vi "tiffU16to2xU8.vi"(10 "U16":u16[][](array[numeric])) -> (2 "Bytes":u8[](array[numeric]))   [LabVIEW 2017, in "LVTiffWriter.lvlib"]
uses:
  LVTiffWriter.lvlib
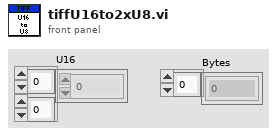
[diagram p1: front panel]
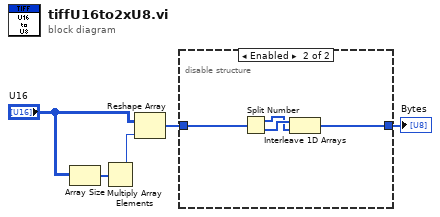
[diagram p0: block diagram]
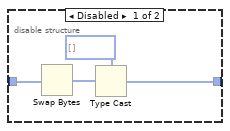
[diagram p2: hidden frame]
diagram:
  n1 = Array Size(array="U16") -> (size(s)=w2:i32[])
  n2 = Multiply Array Elements(1:w2) -> (0:w3:i32)
  n3 = Reshape Array("U16", w3) -> (w1:u16[])
  n4 = disable-structure shown="Enabled" {
    disable-tunnel: [w8 w10] -> w4
    disable-tunnel: w1 -> [w7 w11]
    frame Disabled {
      n5 = Swap Bytes(anything=w7) -> (byte swapped=w6:u16[])
      n6 = Type Cast(type=u8[] [], x=w6) -> (*(type *) &x=w8:u8[])
    }
    frame Enabled {
      n7 = Split Number(x=w11) -> (hi(x)=w12:u8[], lo(x)=w13:u8[])
      n8 = Interleave 1D Arrays(w13, w12) -> (w10:u8[])
    }
  }
  "Bytes" <- w4
